vi "Calc - Y1.vi"(10 "C.39":dbl, 11 "RP1P2":dbl) -> (3 "Y1":dbl)   [LabVIEW 2018, in "Controller (Host).lvlib"]
uses:
  Controller (Host).lvlib
panel:
  out "decimal integer string":string
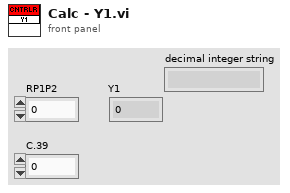
[diagram p1: front panel]
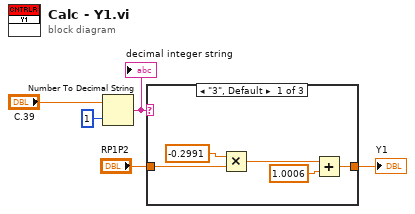
[diagram p0: block diagram]
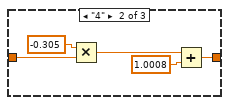
[diagram p2: hidden frame]
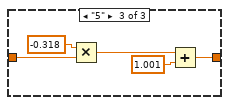
[diagram p3: hidden frame]
diagram:
  n1 = Number To Decimal String(number="C.39", width (-)=i16 1) -> (decimal integer string=w2:string)
  "decimal integer string" <- w2
  n2 = case shown="\"3\", Default" w2 {
    tunnel: "RP1P2" -> [w7 w12 w19]
    tunnel: [w6 w11 w16] -> w5
    frame "3", Default {
      n3 = Multiply(x=-0.2991 ("Default Val"), y=w7) -> (x*y=w9:dbl)
      n4 = Add(x=w9, y=1.0006) -> (x+y=w6:dbl)
    }
    frame "4" {
      n5 = Multiply(x=-0.305 ("Default Val"), y=w12) -> (x*y=w14:dbl)
      n6 = Add(x=w14, y=1.0008) -> (x+y=w11:dbl)
    }
    frame "5" {
      n7 = Multiply(x=-0.318 ("Default Val"), y=w19) -> (x*y=w18:dbl)
      n8 = Add(x=w18, y=1.001) -> (x+y=w16:dbl)
    }
  }
  "Y1" <- w5
